vi "Pre-Run.vi"(8 "error in (no error)":errorcluster, 11 "Actor in":refnum<class "Actor.lvclass">) -> (0 "error out":errorcluster, 3 "Actor out":refnum<class "Actor.lvclass">)   [LabVIEW 2018, in "Actor.lvclass"]
uses:
  Actor.lvclass
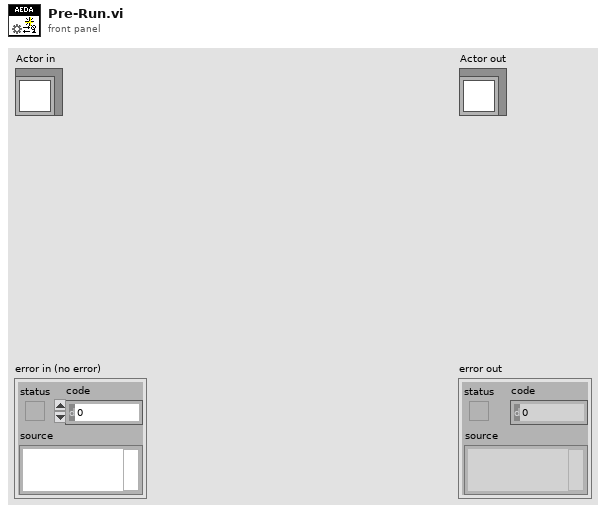
[diagram p1: front panel]
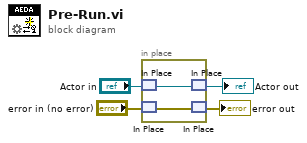
[diagram p0: block diagram]
diagram:
  n1 = in-place {
    n2 = in-place-match #1("Actor in") -> (w6:refnum<class "Actor.lvclass">)
    n3 = in-place-match #2("error in (no error)") -> (w5:errorcluster)
    n4 = in-place-match #1(w6) -> (→"Actor out":refnum<class "Actor.lvclass">)
    n5 = in-place-match #2(w5) -> (→"error out":errorcluster)
  }
